vi "startingTimestamp.get.vi"(8 "error in (no error)":errorcluster, 11 "noManifest in":refnum<class "noManifest.lvclass">) -> (0 "error out":errorcluster, 2 "startingTimestamp":cluster{"seconds":i64, "nanos":i64, "picos":i64}, 3 "noManifest out":refnum<class "noManifest.lvclass">)   [LabVIEW 2020, in "nominal types.lvlib" / "timestampManifest.lvlib" / "noManifest.lvclass"]
uses:
  noManifest.lvclass
  noManifest.lvclass/noManifest.ctl
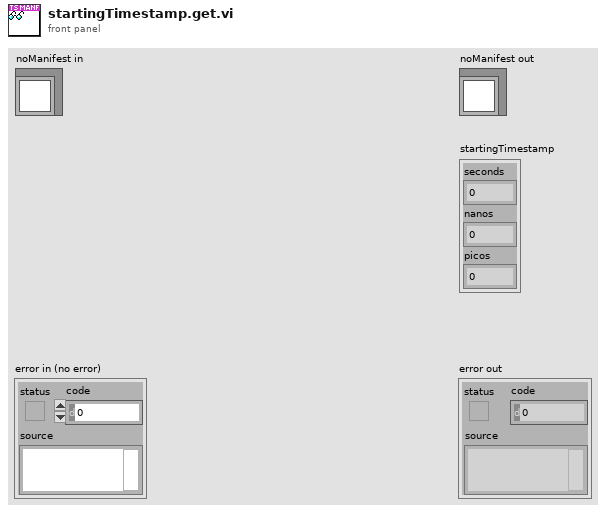
[diagram p1: front panel]
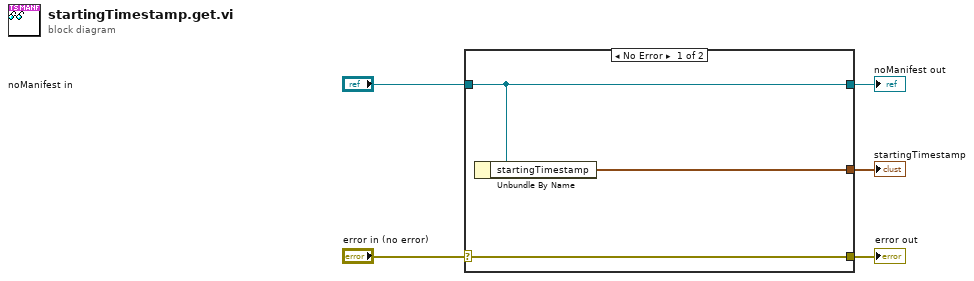
[diagram p0: block diagram]
diagram:
  n1 = case shown="No Error" "error in (no error)" {
    selector: "error in (no error)" -> [w8 w9]
    tunnel: [w8 w9] -> w4
    tunnel: [w7 w10] -> w2
    tunnel: "noManifest in" -> [w7 w10]
    tunnel: [w6 _] -> w1
    frame No Error {
      n2 = Unbundle By Name(w7) -> ("startingTimestamp"=w6:cluster{"seconds":i64, "nanos":i64, "picos":i64})
    }
    frame Error {
    }
  }
  "error out" <- w4
  "noManifest out" <- w2
  "startingTimestamp" <- w1
